vi "CRYStd header find.vi"(10 "Flat data":string, 11 "Main info cluster":T1) -> (3 "Main info cluster out":T1)   [LabVIEW 2013]
uses:
  Control/CRYImp wiz main info.ctl
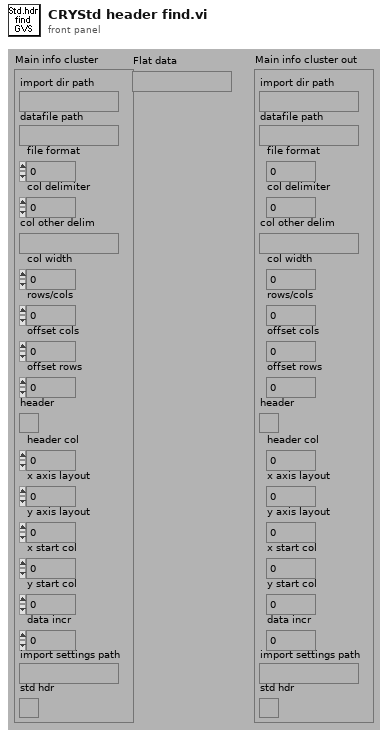
[diagram p1: front panel]
types:
  T1 = typedef "CRYImp wiz main info.ctl" = cluster{"import dir path":path, "datafile path":path, "file format":i32, "col delimiter":i32, "col other delim":string, "col width":i32, "rows/cols":i32, "offset cols":i32, "offset rows":i32, "header":bool, "header col":i32, "x axis layout":i32, "y axis layout":i32, "x start col":i32, "y start col":i32, "data incr":i32, "import settings path":path, "std hdr":bool}
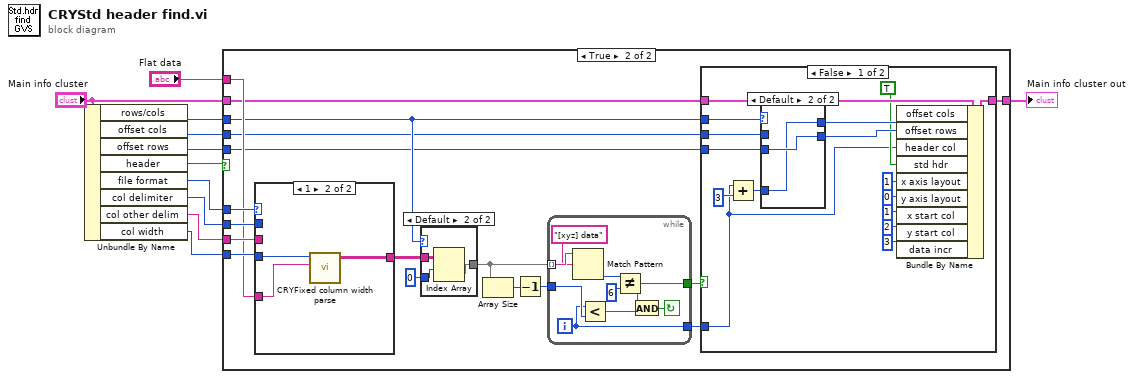
[diagram p0: block diagram]
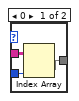
[diagram p5: hidden frame]
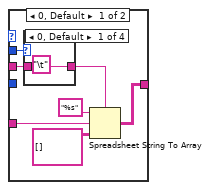
[diagram p6: hidden frame]
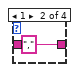
[diagram p7: hidden frame]
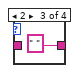
[diagram p8: hidden frame]
diagram:
  n1 = Unbundle By Name("Main info cluster") -> ("rows/cols"=w9:i32, "offset cols"=w8:i32, "offset rows"=w7:i32, "header"=w1:bool, "file format"=w5:i32, "col delimiter"=w4:i32, "col other delim"=w3:string, "col width"=w2:i32)
  n2 = case shown="True" w1 {
    tunnel: "Main info cluster" -> [w12 w17]
    tunnel: [w12 w16] -> w10
    tunnel: w9 -> [_ w15]
    tunnel: w8 -> [_ w14]
    tunnel: w7 -> [_ w13]
    tunnel: "Flat data" -> [_ w25]
    tunnel: w5 -> [_ w29]
    tunnel: w4 -> [_ w28]
    tunnel: w3 -> [_ w27]
    tunnel: w2 -> [_ w26]
    frame False {
    }
    frame True {
      n3 = case shown="1" w29 {
        tunnel: w28 -> [w72 _]
        tunnel: w27 -> [w71 _]
        tunnel: w25 -> [w67 w78]
        tunnel: w26 -> [_ w79]
        tunnel: [w66 w77] -> w23
        frame 0, Default {
          n4 = case shown="0, Default" w72 {
            tunnel: w71 -> [_ _ _ w76]
            tunnel: ["\t" "," " " w76] -> w68
            frame 0, Default {
            }
            frame 1 {
            }
            frame 2 {
            }
            frame 3 {
            }
          }
          n5 = Spreadsheet String To Array(delimiter (Tab)=w68, format string="%s", spreadsheet string=w67, array type (2D Dbl)=string[][] []) -> (array=w66:string[][])
        }
        frame 1 {
          n6 = call "CRYFixed column width parse.vi"("Data string"=w78, "Fixed column width"=w79) -> ("2D string array"=w77:string[][])  [unwired: 9 in]
        }
      }
      n7 = case shown="Default" w15 {
        tunnel: 0 ("Index") -> [w62 w65]
        tunnel: w23 -> [w61 w64]
        tunnel: [w60 w63] -> w22
        frame 0 {
          n8 = Index Array(array=w61, index (col)=w62) -> (element=w60:string[])  [unwired: 1 in]
        }
        frame Default {
          n9 = Index Array(array=w64, index (row)=w65) -> (element=w63:string[])  [unwired: 1 in]
        }
      }
      n10 = Array Size(array=w22) -> (size(s)=w21:i32)
      n11 = Decrement(x=w21) -> (x-1=w20:i32)
      n12 = while {
        tunnel: [w30] -> w18
        tunnel: [w32] -> w19
        tunnel: w20 -> [w38]
        tunnel: w22 -> [w37] mode=indexing
        i -> [w30]
        stop <- w31 continue-if-true
        n13 = Match Pattern(string=w37, regular expression="[xyz] data") -> (offset past match=w35:i32)  [unwired: 4 out]
        n14 = Less?(x=w30, y=w38) -> (x < y?=w33:bool)
        n15 = Not Equal?(x=w35, y=6) -> (x != y?=w32:bool)
        n16 = And(x=w32, y=w33) -> (x .and. y?=w31:bool)
      }
      n17 = case shown="False" w19 {
        tunnel: w18 -> [w44 _]
        tunnel: [w53 w59] -> w16
        tunnel: w17 -> [w54 w59]
        tunnel: w15 -> [w51 _]
        tunnel: w14 -> [w47 _]
        tunnel: w13 -> [w46 _]
        frame False {
          n18 = Add(x=w44, y=3 ("Bundle Element")) -> (x+y=w49:i32)
          n19 = case shown="Default" w51 {
            tunnel: [w56 w58] -> w50
            tunnel: w49 -> [w56 w57]
            tunnel: [w55 w57] -> w48
            tunnel: w47 -> [w55 _]
            tunnel: w46 -> [_ w58]
            frame 0 {
            }
            frame Default {
            }
          }
          n20 = Bundle By Name(cluster=w54, "offset cols"=w48, "offset rows"=w50, "header col"=w44, "std hdr"=TRUE, "x axis layout"=1 ("Bundle Element"), "y axis layout"=0 ("Bundle Element"), "x start col"=1 ("Bundle Element"), "y start col"=2 ("Bundle Element"), "data incr"=3 ("Bundle Element")) -> (w53:T1)
        }
        frame True {
        }
      }
    }
  }
  "Main info cluster out" <- w10
